vi "dynamic parse test.vi"() -> ()   [LabVIEW 2015]
uses:
  API/JSON Document Class/JSON Document.lvclass
panel:
  in  "JSON String":string="true"
  out "Table Control":string[][](table)
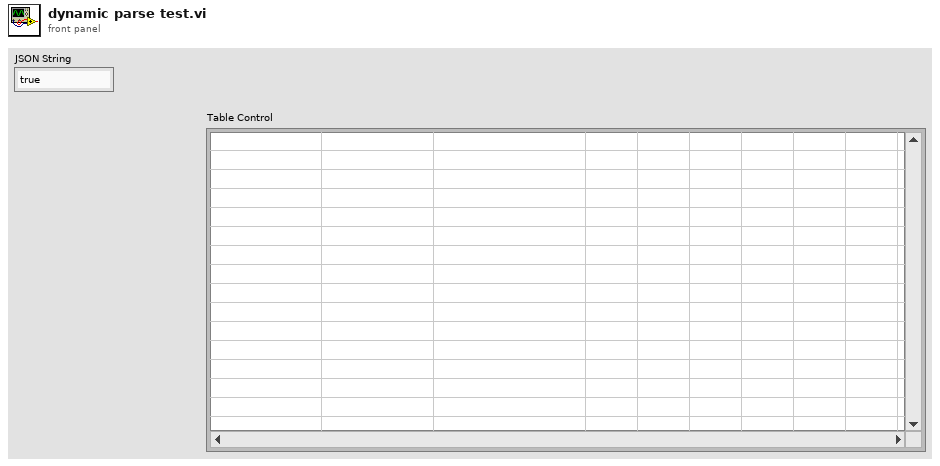
[diagram p1: front panel]
types:
  T1 = cluster{"default?":string, "value":string, "type":string}
  T2 = cluster{"default?":string, "value":string, "type":string}[]
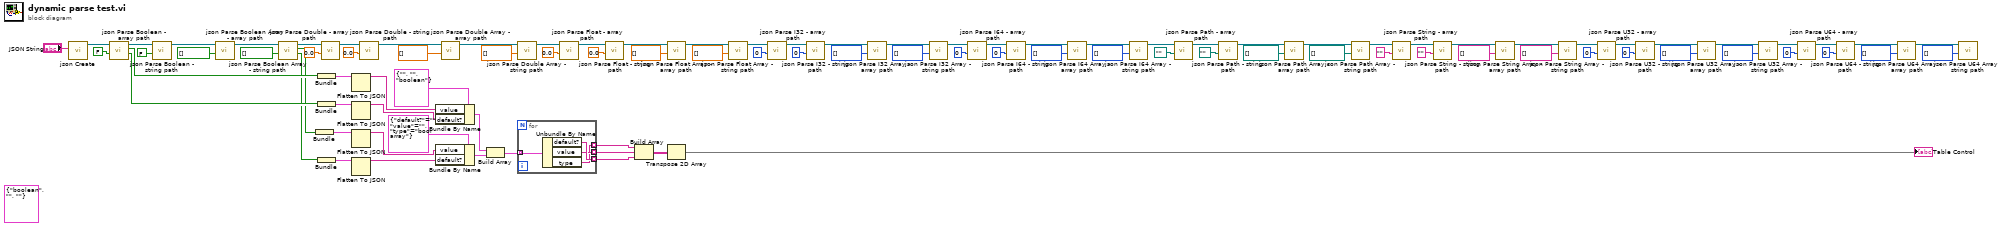
[diagram p0: block diagram]
diagram:
  (unwired) T1 {"default?"="boolean", "value"="", "type"=""} ("table row")
  n1 = call "json Create.vi"("JSON String"="JSON String") -> ("JSON Document out"=w42:refnum<class "JSON Document.lvclass">)  [unwired: 9 in, 1 out]
  n2 = call "json Parse Boolean - array path.vi"("default"=FALSE, "JSON Document in"=w42) -> ("defaulted?"=w19:bool, "value"=w21:bool, "JSON Document out"=w95:refnum<class "JSON Document.lvclass">)  [unwired: 6 in, 1 out]
  n3 = call "json Parse Boolean - string path.vi"("default"=FALSE, "JSON Document in"=w95) -> ("JSON Document out"=w94:refnum<class "JSON Document.lvclass">)  [unwired: 6 in, 3 out]
  n4 = call "json Parse Boolean Array - array path.vi"("default"=bool[] [], "JSON Document in"=w94) -> ("JSON Document out"=w93:refnum<class "JSON Document.lvclass">)  [unwired: 5 in, 4 out]
  n5 = call "json Parse Boolean Array - string path.vi"("default"=bool[] [], "JSON Document in"=w93) -> ("defaulted?"=w11:bool, "value"=w12:bool[], "JSON Document out"=w92:refnum<class "JSON Document.lvclass">)  [unwired: 5 in, 2 out]
  n6 = Bundle("value"=w12) -> (w13:cluster{"value":bool[]})  [unwired: 1 in]
  n7 = Bundle("value"=w21) -> (w22:cluster{"value":bool})  [unwired: 1 in]
  n8 = Bundle("defaulted?"=w19) -> (w20:cluster{"defaulted?":bool})  [unwired: 1 in]
  n9 = Bundle("defaulted?"=w11) -> (w14:cluster{"defaulted?":bool})  [unwired: 1 in]
  n10 = call "json Parse Double - array path.vi"("default"=0.0, "JSON Document in"=w92) -> ("JSON Document out"=w91:refnum<class "JSON Document.lvclass">)  [unwired: 6 in, 3 out]
  n11 = Flatten To JSON(anything=w22) -> (JSON string=w17:string)  [unwired: 2 in, 1 out]
  n12 = Flatten To JSON(anything=w20) -> (JSON string=w18:string)  [unwired: 2 in, 1 out]
  n13 = Flatten To JSON(anything=w13) -> (JSON string=w16:string)  [unwired: 2 in, 1 out]
  n14 = Flatten To JSON(anything=w14) -> (JSON string=w15:string)  [unwired: 2 in, 1 out]
  n15 = call "json Parse Double - string path.vi"("default"=0.0, "JSON Document in"=w91) -> ("JSON Document out"=w90:refnum<class "JSON Document.lvclass">)  [unwired: 6 in, 3 out]
  n16 = Bundle By Name(cluster=T1 {"default?"="", "value"="", "type"="boolean"} ("table row"), "value"=w17, "default?"=w18) -> (w9:T1)
  n17 = Bundle By Name(cluster=T1 {"default?"="", "value"="", "type"="bool array"} ("input cluster"), "value"=w16, "default?"=w15) -> (w8:T1)
  n18 = call "json Parse Double Array - array path.vi"("default"=dbl[] [], "JSON Document in"=w90) -> ("JSON Document out"=w89:refnum<class "JSON Document.lvclass">)  [unwired: 5 in, 4 out]
  n19 = Build Array(w9, w8) -> (w7:T2)
  n20 = call "json Parse Double Array - string path.vi"("default"=dbl[] [], "JSON Document in"=w89) -> ("JSON Document out"=w88:refnum<class "JSON Document.lvclass">)  [unwired: 5 in, 4 out]
  n21 = for {
    tunnel: w7 -> [w99] mode=indexing
    tunnel: [w98] -> w4 mode=indexing
    tunnel: [w97] -> w5 mode=indexing
    tunnel: [w96] -> w6 mode=indexing
    n22 = Unbundle By Name(w99) -> ("default?"=w98:string, "value"=w97:string, "type"=w96:string)
  }
  n23 = call "json Parse Float - array path.vi"("default"=sgl 0.0, "JSON Document in"=w88) -> ("JSON Document out"=w87:refnum<class "JSON Document.lvclass">)  [unwired: 6 in, 3 out]
  n24 = call "json Parse Float - string path.vi"("default"=sgl 0.0, "JSON Document in"=w87) -> ("JSON Document out"=w86:refnum<class "JSON Document.lvclass">)  [unwired: 6 in, 3 out]
  n25 = Build Array(w6, w5, w4) -> (w3:string[][])
  n26 = call "json Parse Float Array - array path.vi"("default"=sgl[] [], "JSON Document in"=w86) -> ("JSON Document out"=w85:refnum<class "JSON Document.lvclass">)  [unwired: 5 in, 4 out]
  n27 = Transpose 2D Array(2D array=w3) -> (transposed array=→"Table Control":string[][])
  n28 = call "json Parse Float Array - string path.vi"("default"=sgl[] [], "JSON Document in"=w85) -> ("JSON Document out"=w84:refnum<class "JSON Document.lvclass">)  [unwired: 5 in, 4 out]
  n29 = call "json Parse I32 - array path.vi"("default"=0, "JSON Document in"=w84) -> ("JSON Document out"=w83:refnum<class "JSON Document.lvclass">)  [unwired: 6 in, 3 out]
  n30 = call "json Parse I32 - string path.vi"("default"=0, "JSON Document in"=w83) -> ("JSON Document out"=w82:refnum<class "JSON Document.lvclass">)  [unwired: 6 in, 3 out]
  n31 = call "json Parse I32 Array - array path.vi"("default"=i32[] [], "JSON Document in"=w82) -> ("JSON Document out"=w81:refnum<class "JSON Document.lvclass">)  [unwired: 5 in, 4 out]
  n32 = call "json Parse I32 Array - string path.vi"("default"=i32[] [], "JSON Document in"=w81) -> ("JSON Document out"=w80:refnum<class "JSON Document.lvclass">)  [unwired: 5 in, 4 out]
  n33 = call "json Parse I64 - array path.vi"("default"=i64 0, "JSON Document in"=w80) -> ("JSON Document out"=w41:refnum<class "JSON Document.lvclass">)  [unwired: 6 in, 3 out]
  n34 = call "json Parse I64 - string path.vi"("default"=i64 0, "JSON Document in"=w41) -> ("JSON Document out"=w40:refnum<class "JSON Document.lvclass">)  [unwired: 6 in, 3 out]
  n35 = call "json Parse I64 Array - array path.vi"("default"=i64[] [], "JSON Document in"=w40) -> ("JSON Document out"=w39:refnum<class "JSON Document.lvclass">)  [unwired: 5 in, 4 out]
  n36 = call "json Parse I64 Array - string path.vi"("default"=i64[] [], "JSON Document in"=w39) -> ("JSON Document out"=w38:refnum<class "JSON Document.lvclass">)  [unwired: 5 in, 4 out]
  n37 = call "json Parse Path - array path.vi"("default"=path "", "JSON Document in"=w38) -> ("JSON Document out"=w37:refnum<class "JSON Document.lvclass">)  [unwired: 6 in, 3 out]
  n38 = call "json Parse Path - string path.vi"("default"=path "", "JSON Document in"=w37) -> ("JSON Document out"=w36:refnum<class "JSON Document.lvclass">)  [unwired: 6 in, 3 out]
  n39 = call "json Parse Path Array - array path.vi"("default"=path[] [], "JSON Document in"=w36) -> ("JSON Document out"=w35:refnum<class "JSON Document.lvclass">)  [unwired: 5 in, 4 out]
  n40 = call "json Parse Path Array - string path.vi"("default"=path[] [], "JSON Document in"=w35) -> ("JSON Document out"=w34:refnum<class "JSON Document.lvclass">)  [unwired: 5 in, 4 out]
  n41 = call "json Parse String - array path.vi"("default"="", "JSON Document in"=w34) -> ("JSON Document out"=w33:refnum<class "JSON Document.lvclass">)  [unwired: 6 in, 3 out]
  n42 = call "json Parse String - string path.vi"("default"="", "JSON Document in"=w33) -> ("JSON Document out"=w79:refnum<class "JSON Document.lvclass">)  [unwired: 6 in, 3 out]
  n43 = call "json Parse String Array - array path.vi"("default"=string[] [], "JSON Document in"=w79) -> ("JSON Document out"=w32:refnum<class "JSON Document.lvclass">)  [unwired: 5 in, 4 out]
  n44 = call "json Parse String Array - string path.vi"("default"=string[] [], "JSON Document in"=w32) -> ("JSON Document out"=w31:refnum<class "JSON Document.lvclass">)  [unwired: 5 in, 4 out]
  n45 = call "json Parse U32 - array path.vi"("default"=u32 0, "JSON Document in"=w31) -> ("JSON Document out"=w30:refnum<class "JSON Document.lvclass">)  [unwired: 6 in, 3 out]
  n46 = call "json Parse U32 - string path.vi"("default"=u32 0, "JSON Document in"=w30) -> ("JSON Document out"=w29:refnum<class "JSON Document.lvclass">)  [unwired: 6 in, 3 out]
  n47 = call "json Parse U32 Array - array path.vi"("default"=u32[] [], "JSON Document in"=w29) -> ("JSON Document out"=w28:refnum<class "JSON Document.lvclass">)  [unwired: 5 in, 4 out]
  n48 = call "json Parse U32 Array - string path.vi"("default"=u32[] [], "JSON Document in"=w28) -> ("JSON Document out"=w27:refnum<class "JSON Document.lvclass">)  [unwired: 5 in, 4 out]
  n49 = call "json Parse U64 - array path.vi"("default"=u64 0, "JSON Document in"=w27) -> ("JSON Document out"=w26:refnum<class "JSON Document.lvclass">)  [unwired: 6 in, 3 out]
  n50 = call "json Parse U64 - string path.vi"("default"=u64 0, "JSON Document in"=w26) -> ("JSON Document out"=w78:refnum<class "JSON Document.lvclass">)  [unwired: 6 in, 3 out]
  n51 = call "json Parse U64 Array - array path.vi"("default"=u64[] [], "JSON Document in"=w78) -> ("JSON Document out"=w25:refnum<class "JSON Document.lvclass">)  [unwired: 5 in, 4 out]
  n52 = call "json Parse U64 Array - string path.vi"("default"=u64[] [], "JSON Document in"=w25) -> ()  [unwired: 5 in, 5 out]
